vi "Actor Core.vi"(8 "error in":errorcluster, 11 "Series Actor in":refnum<class "Series Actor.lvclass">) -> (0 "error out":errorcluster, 3 "Actor out":refnum<class "Actor.lvclass">)   [LabVIEW 2024, in "Series Actor.lvlib" / "Series Actor.lvclass"]
doc: "(<B>Filename</B>: Actor Framework.lvlib:Actor.lvclass:Actor Core.vi)\n\nReceives messages to the actor, reacts to them, and initiates any error handling that may shut the actor down.\n\nDescendant classes may override this VI to append parallel tasks for the actor to complete while it handles messages. Overrides use the Call Parent Class Method node."
uses:
  Series Actor.lvclass
  <vilib>/ActorFramework/Actor/Actor.lvclass
  <vilib>/MGI/Panel Manager/Panel Actor/Panel Actor/Panel Actor.lvclass
  Series Actor.lvclass/Series Actor.ctl
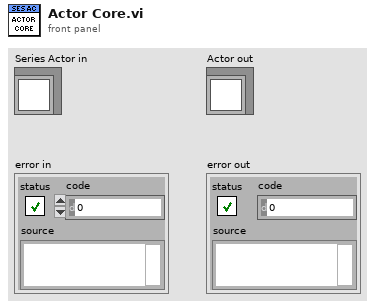
[diagram p1: front panel]
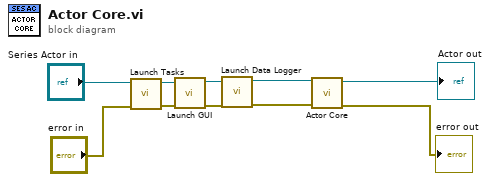
[diagram p0: block diagram]
diagram:
  n1 = call "Launch Tasks.vi"("error in"="error in", "Series Actor in"="Series Actor in") -> ("error out"=w7:errorcluster, "Series Actor out"=w4:refnum<class "Series Actor.lvclass">)  [unwired: 8 in]
  n2 = call-dynamic "Launch GUI.vi"("error in"=w7, "Series Actor in"=w4) -> ("error out"=w8:errorcluster, "Series Actor out"=w3:refnum<class "Series Actor.lvclass">)  [unwired: 8 in]
  n3 = call "Launch Data Logger.vi"("error in"=w8, "Series Actor in"=w3) -> ("error out"=w1:errorcluster, "Series Actor out"=w2:refnum<class "Series Actor.lvclass">)  [unwired: 8 in]
  n4 = call-parent "Actor Core.vi"("error in"=w1, "Panel Actor in"=w2) -> ("error out"=→"error out":errorcluster, "Actor out"=→"Actor out":refnum<class "Actor.lvclass">)  [unwired: 8 in]
